vi "gen random emmiters.vi"(10 "rand limits":T14={"DOA range "={1634128.9560392164, 2964508.639841233}, "modulation depth"={67532.40039072247, 205475.5312375231}, "num of hoopers"=10, "num of frequncyes"={2, 1}, "QPSK"=TRUE, "BPSK"=TRUE, "LFM"=TRUE, "CW"=TRUE, "     f band range"={-77296466.97388633, 78525345.62211981}, "D.C range"={0.5407066052227343, 0.5038402457757296}, "hop rate range"={2.0915680786684536, 3.1385684721559217}, "span range "={1634128.9560392164, 2964508.639841233}, "amp range"={-21.121351766513058, -25.88325652841782}, "start time (sec)"=0.0, "end time (sec)"=50.0} {"start time (sec)" format="%#_13g"; "amp range" scale=0.0..-50.0 scale format="%#_g dB"; "span range" scale=1000000.0..30000000.0 scale format="%#_6p Hz"; "hop rate range" scale=1.0..3000.0 scale format="%#_6p"; "D.C range" scale=0.0..1.0; "f band range" scale=-1600000000.0..1600000000.0 scale format="%#_6p Hz"; "num of frequncyes" scale=1.0..300.0; "num of hoopers" scale=0.0..200.0; "modulation depth" scale=10000.0..30000000.0 scale format="%#_6p Hz"; "DOA range" scale=0.0..360.0 scale format="%#_6p deg"}, 11 "secnario config":T1={"devicess 2"=["IF_transiver_1", "IF_transiver_2"], "file paths"=[path "C:/Users/PXIe8108_Demo/Documents/CHAIM DATA/chaim/5785_sync_for_elbit/data/pdw_test_file.tdms", path "C:/Users/PXIe8108_Demo/Documents/CHAIM DATA/chaim/5785_sync_for_elbit/data/pdw_test_file.tdms", path "C:/Users/PXIe8108_Demo/Documents/CHAIM DATA/chaim/5785_sync_for_elbit/data/pdw_test_file.tdms", path "C:/Users/PXIe8108_Demo/Documents/CHAIM DATA/chaim/5785_sync_for_elbit/data/pdw_test_file.tdms"], "buffer size"=524288, "Fs  FPGA"=200000000.0, "SPC"=16.0, "center frequency (Hz) "=1000000000.0, "t clock ref"=[], "fpga rfe"=[], "tdms refs"=[], "niUsrpRio Session (out)"={"FPGA Interface"=refnum, "RIO Interface Number"=0, "Data Clock Rate"=0, "FPGA Data Clock Rate"=0, "Global Settings Register Bus"=refnum, "Radio 0 Settings Register Bus"=refnum, "Radio 1 Settings Register Bus"=refnum, "Radio Settings Bus Semaphore"=refnum, "DB Queues"=[], "Characterization Data Valid?"=FALSE, "EEPROM Header"={"Checksum"=0, "Product Code"=0, "Hardware Current Version"=0, "Hardware Oldest Compatible Version"=0, "EEPROM Map Current Version"=0, "EEPROM Map Oldest Compatible Version"=0, "User Password"="", "Pointer to Factory Header"=0, "Pointer to User Header"=0, "Recommended Interval"=0, "Number of Reserved Bytes"=9, "Number of Daughterboards"=0, "Daughterboard IDs"=[], "Daughterboard Serial Numbers"=[]}, "Device Data Header"={"Checksum"=0, "Number of Channels"=0, "Number of Gain Settings"=[], "Pointer to Characterization Data"=[], "Number of Reserved Bytes"=27, "Number of Frequencies"=[]}, "EEPROM Characterization Header"={"Checksum"=0, "Date"=timestamp(0 s since 1904-01-01), "Temperature"=0.0, "Misc. Info"="", "Pointer to Device Data Header"=0, "Number of Reserved Bytes"=28}, "Characterization Data"=[], "FPGA Current Version"=0, "FPGA Oldest Compatible Version"=0, "Fixed Logic Current Version"=0, "Fixed Logic Oldest Compatible Version"=0, "FPGA Radio Settings Bus Current Version"=0, "FPGA Radio Settings Bus Oldest Compatible Version"=0, "FPGA Board Config Current Version"=0, "FPGA Board Config Oldest Compatible Version"=0, "Daughterboard Clock Rate"=0, "daughterboard configuration session handles"=[]}, "RF gain "=10, "mode"=0, "vst_device"=[], "IQ_rare_p2p"=200000000.0, "stream sesion P2P"=[]} {"mode" scale=0.0..2.0; "RF gain" min=0 max=31 step=1; "niUsrpRio Session (out)"."Daughterboard Clock Rate" format="%#.3pHz"; "niUsrpRio Session (out)"."FPGA Data Clock Rate" format="%#.3pHz"; "niUsrpRio Session (out)"."Data Clock Rate" format="%#.3pHz"; "niUsrpRio Session (out)"."Characterization Data"."Frequencies [Hz]" format="%#_6p"; "niUsrpRio Session (out)"."EEPROM Characterization Header"."Pointer to Device Data Header" format="%x"; "niUsrpRio Session (out)"."EEPROM Characterization Header"."Checksum" format="%x"; "niUsrpRio Session (out)"."Device Data Header"."Pointer to Characterization Data" format="%x"; "niUsrpRio Session (out)"."Device Data Header"."Checksum" format="%x"; "niUsrpRio Session (out)"."EEPROM Header"."Pointer to User Header" format="%x"; "niUsrpRio Session (out)"."EEPROM Header"."Pointer to Factory Header" format="%x"; "niUsrpRio Session (out)"."EEPROM Header"."Product Code" format="%x"; "niUsrpRio Session (out)"."EEPROM Header"."Checksum" format="%x"; "center frequency (Hz)" format="%#.8p"; "buffer size" step=512}) -> (3 "Array":T12[](array[typedef]) {"t end" format="%#_3p"; "t start" format="%#_3p"; "DOA" format="%#_3p"; "mod depth" format="%#_3p"})   [LabVIEW 2021]
uses:
  random_limits.ctl
  emitter params.ctl
  mode_type.ctl
  secnario config.ctl
  <vilib>/userdefined/High Color/nirio_resource_hc.ctl
  <instrlib>/niUsrpRio/Config/v1/Host/Public/niUsrpRio Session.ctl
  <instrlib>/_niInstr/Register Bus/v0/Host/Public/Register Bus Session.ctl
  <instrlib>/_niInstr/Register Bus/v0/Host/Private/Session Data.ctl
  <instrlib>/niUsrpRio/Config/v1/Host/Private/DB Queue Reference.ctl
  <instrlib>/niUsrpRio/Config/v1/Host/Private/Daughterboard Data.ctl
  <instrlib>/niUsrpRio/Config/v1/Host/Private/ATR state data.ctl
  <instrlib>/niUsrpRio/Config/v1/Host/Private/Antenna Configuration.ctl
  <instrlib>/niUsrpRio/Config/v1/Host/Private/CPLD Power Mode.ctl
  <instrlib>/niUsrpRio/Config/v1/Host/Public/EEPROM Header.ctl
  <instrlib>/niUsrpRio/Config/v1/Host/Public/EEPROM Device Data Header.ctl
  <instrlib>/niUsrpRio/Config/v1/Host/Public/EEPROM Characterization Header.ctl
  <instrlib>/niUsrpRio/Config/v1/Host/Public/Characterization Data.ctl
  <instrlib>/niUsrpRio/Config/v1/Host/Public/IQ Imbalance.ctl
  <vilib>/numeric/Random Number (Range) DBL.vi
  <vilib>/numeric/Random Number (Range) U64.vi
  <vilib>/numeric/sub_Random U32.vi
  <instrlib>/_niInstr/Register Bus/v0/Host/niInstr Register Bus v0 Host.lvlib
  <instrlib>/niUsrpRio/Config/v1/Host/niUsrpRio Config v1 Host.lvlib
panel:
  # "available modulations:"
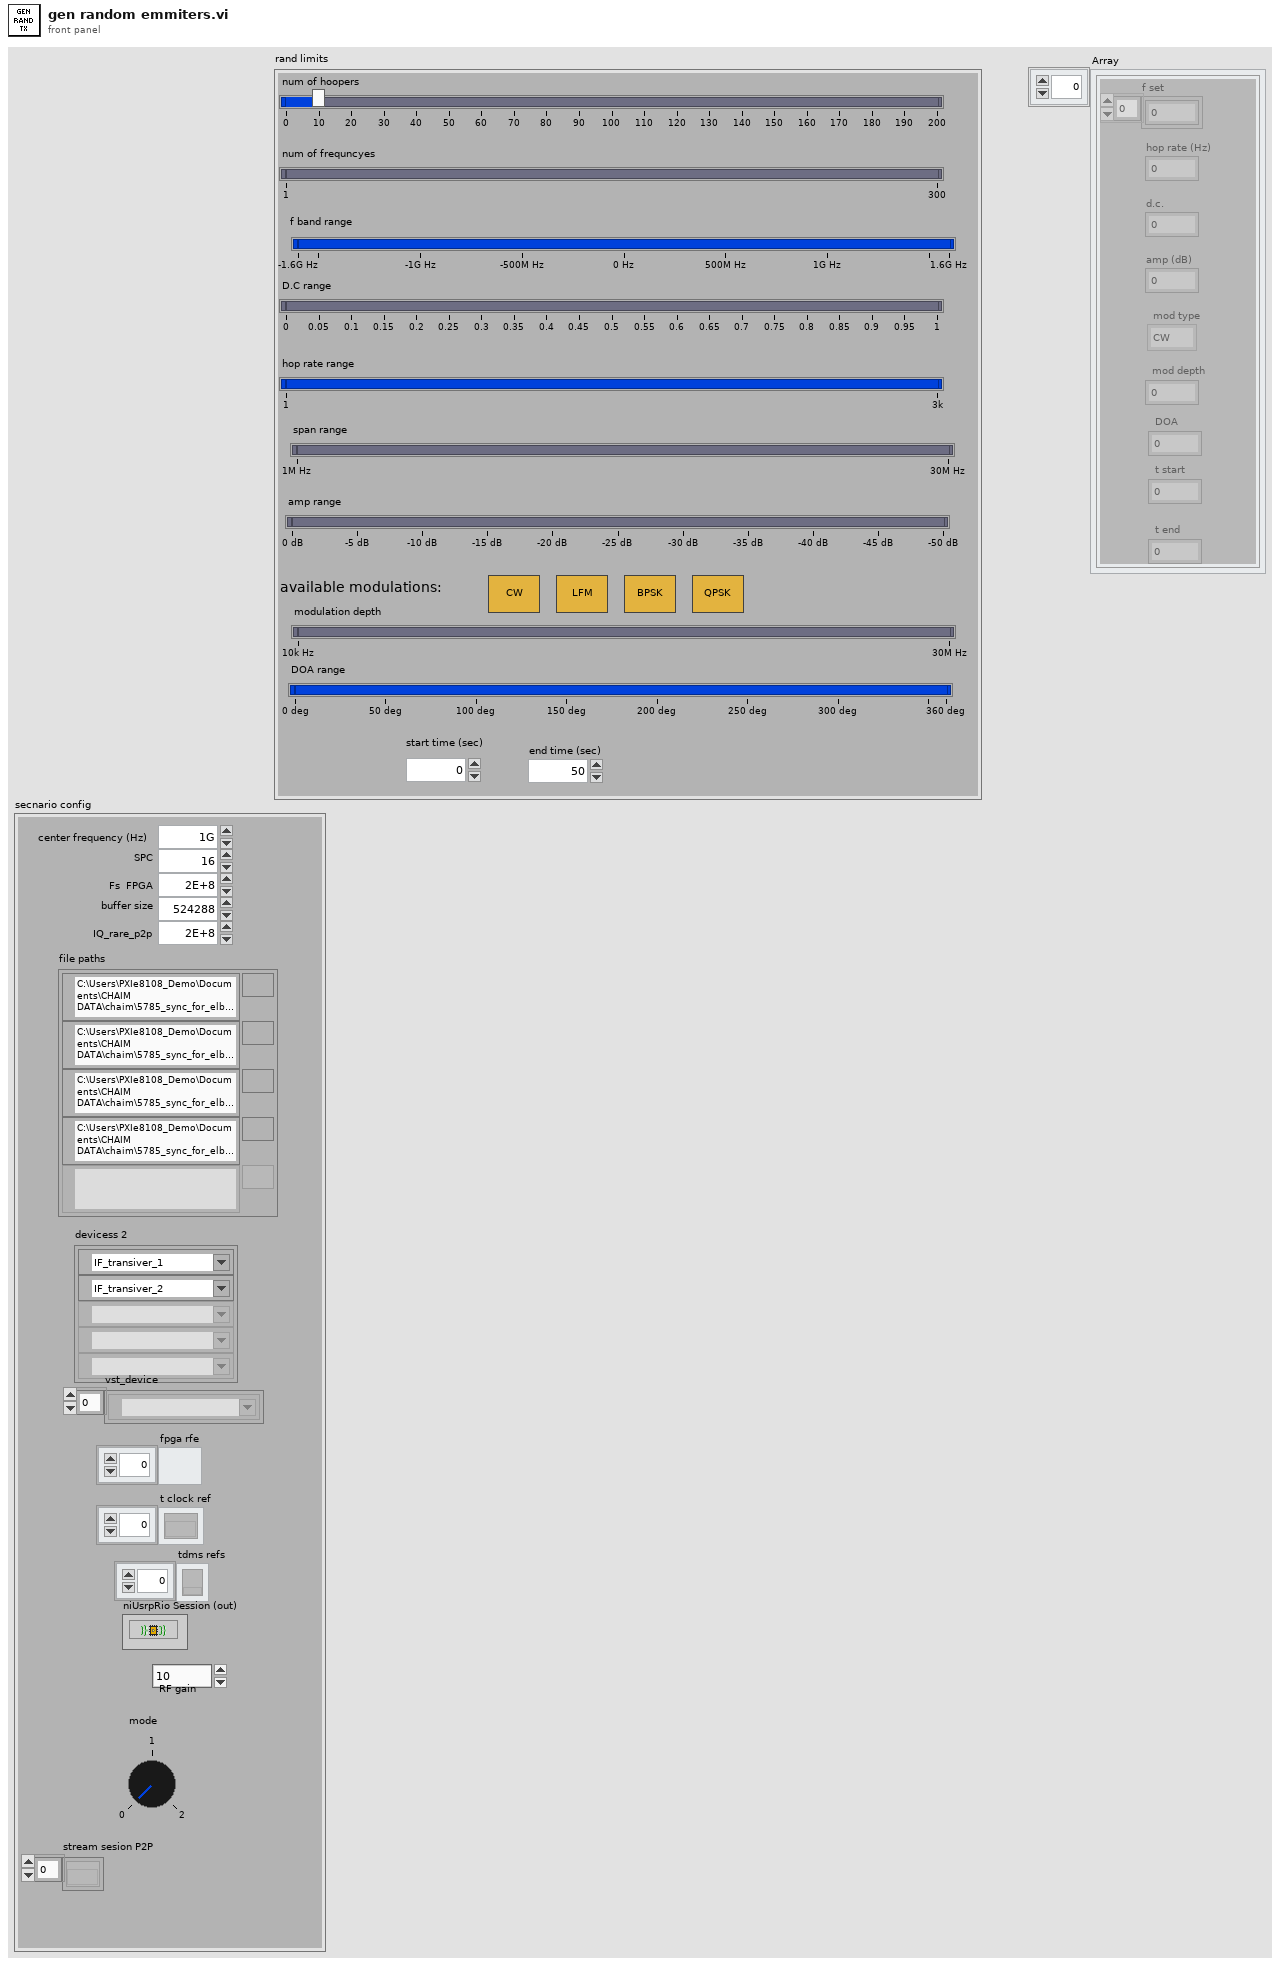
[diagram p1: front panel]
types:
  T1 = typedef "secnario config.ctl" = cluster{"devicess 2":T2[], "file paths":path[], "buffer size":u32, "Fs  FPGA":dbl, "SPC":dbl, "center frequency (Hz) ":dbl, "t clock ref":refnum<k20>[], "fpga rfe":refnum<k20>[], "tdms refs":refnum<k34>[], "niUsrpRio Session (out)":T3, "RF gain ":i32, "mode":u8, "vst_device":refnum<k15>[], "IQ_rare_p2p":dbl, "stream sesion P2P":refnum<k20>[]}
  T2 = typedef "nirio_resource_hc.ctl" = tag
  T3 = typedef "niUsrpRio Config v1 Host.lvlib/niUsrpRio Session.ctl" = cluster{"FPGA Interface":refnum<k20>, "RIO Interface Number":u32, "Data Clock Rate":u32, "FPGA Data Clock Rate":u32, "Global Settings Register Bus":T4, "Radio 0 Settings Register Bus":T4, "Radio 1 Settings Register Bus":T4, "Radio Settings Bus Semaphore":T5, "DB Queues":T6[], "Characterization Data Valid?":bool, "EEPROM Header":T7, "Device Data Header":T8, "EEPROM Characterization Header":T9, "Characterization Data":T10[], "FPGA Current Version":u32, "FPGA Oldest Compatible Version":u32, "Fixed Logic Current Version":u32, "Fixed Logic Oldest Compatible Version":u32, "FPGA Radio Settings Bus Current Version":u32, "FPGA Radio Settings Bus Oldest Compatible Version":u32, "FPGA Board Config Current Version":u32, "FPGA Board Config Oldest Compatible Version":u32, "Daughterboard Clock Rate":u32, "daughterboard configuration session handles":u64[]}
  T4 = typedef "niInstr Register Bus v0 Host.lvlib/Register Bus Session.ctl" = refnum<queue>
  T5 = typedef "Semaphore RefNum" = refnum<k1>
  T6 = typedef "niUsrpRio Config v1 Host.lvlib/DB Queue Reference.ctl" = refnum<queue>
  T7 = typedef "niUsrpRio Config v1 Host.lvlib/EEPROM Header.ctl" = cluster{"Checksum":u32, "Product Code":u16, "Hardware Current Version":u16, "Hardware Oldest Compatible Version":u16, "EEPROM Map Current Version":u16, "EEPROM Map Oldest Compatible Version":u16, "User Password":string, "Pointer to Factory Header":u32, "Pointer to User Header":u32, "Recommended Interval":u16, "Number of Reserved Bytes":i32, "Number of Daughterboards":u8, "Daughterboard IDs":u16[], "Daughterboard Serial Numbers":string[]}
  T8 = typedef "niUsrpRio Config v1 Host.lvlib/EEPROM Device Data Header.ctl" = cluster{"Checksum":u32, "Number of Channels":u8, "Number of Gain Settings":u16[], "Pointer to Characterization Data":u32[], "Number of Reserved Bytes":i32, "Number of Frequencies":u16[]}
  T9 = typedef "niUsrpRio Config v1 Host.lvlib/EEPROM Characterization Header.ctl" = cluster{"Checksum":u32, "Date":timestamp, "Temperature":sgl, "Misc. Info":string, "Pointer to Device Data Header":u32, "Number of Reserved Bytes":i32}
  T10 = typedef "niUsrpRio Config v1 Host.lvlib/Characterization Data.ctl" = cluster{"Gains[dB]":dbl[], "Frequencies [Hz]":dbl[], "IQ Imbalance Table":T11[], "Measured Gains[dB]":dbl[][]}
  T11 = typedef "niUsrpRio Config v1 Host.lvlib/IQ Imbalance.ctl" = cluster{"Gain Imbalance [linear]":dbl, "Phase Imbalance [radians]":dbl, "Offset":cdb}
  T12 = typedef "emitter params.ctl" = cluster{"f set":dbl[], "hop rate (Hz)":dbl, "d.c.":dbl, "amp (dB)":dbl, "mod type":T13, "mod depth":dbl, "DOA":dbl, "t start":dbl, "t end":dbl}
  T13 = typedef "mode_type.ctl" = enum8{"CW", "NC - CW", "NC - cw", "LFM", "BPSK", "QPSK"}
  T14 = typedef "random_limits.ctl" = cluster{"DOA range ":cluster{dbl, dbl}, "modulation depth":cluster{dbl, dbl}, "num of hoopers":i32, "num of frequncyes":cluster{i32, i32}, "QPSK":bool, "BPSK":bool, "LFM":bool, "CW":bool, "     f band range":cluster{dbl, dbl}, "D.C range":cluster{dbl, dbl}, "hop rate range":cluster{dbl, dbl}, "span range ":cluster{dbl, dbl}, "amp range":cluster{dbl, dbl}, "start time (sec)":dbl, "end time (sec)":dbl}
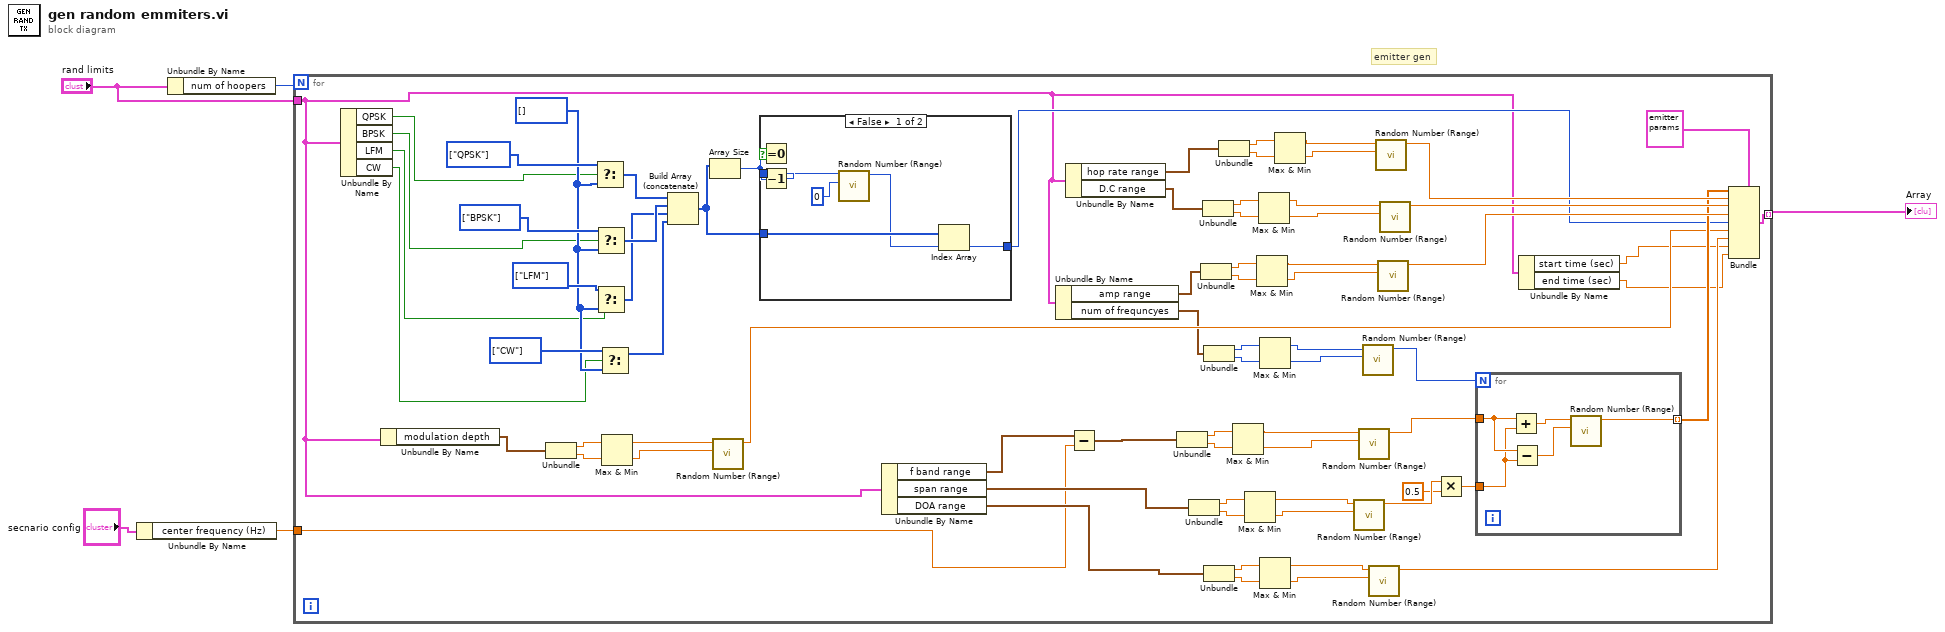
[diagram p0: block diagram]
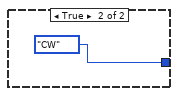
[diagram p2: hidden frame]
diagram:
  # "emitter gen"
  n1 = Unbundle By Name("secnario config") -> ("center frequency (Hz)"=w1:dbl)
  n2 = Unbundle By Name("rand limits") -> ("num of hoopers"=w4:i32)
  n3 = for {
    N: w4 -> [_]
    tunnel: [w72] -> w5 mode=indexing
    tunnel: "rand limits" -> [w10]
    tunnel: w1 -> [w7]
    w32 = T13[] [enum."QPSK"] items=["CW", "NC - CW", "NC - cw", "LFM", "BPSK", "QPSK"]
    w28 = T13[] [] items=["CW", "NC - CW", "NC - cw", "LFM", "BPSK", "QPSK"]
    w31 = T13[] [enum."BPSK"] items=["CW", "NC - CW", "NC - cw", "LFM", "BPSK", "QPSK"]
    w30 = T13[] [enum."LFM"] items=["CW", "NC - CW", "NC - cw", "LFM", "BPSK", "QPSK"]
    w29 = T13[] [enum."CW"] items=["CW", "NC - CW", "NC - cw", "LFM", "BPSK", "QPSK"]
    n4 = Unbundle By Name(w10) -> ("QPSK"=w22:bool, "BPSK"=w21:bool, "LFM"=w20:bool, "CW"=w19:bool)
    n5 = Unbundle By Name(w10) -> ("modulation depth"=w9:cluster{dbl, dbl})
    n6 = Unbundle(w9) -> (w46:dbl, w45:dbl)
    n7 = Select(t=w32, s=w22, f=w28) -> (s? t:f=w42:T13[])
    n8 = Select(t=w31, s=w21, f=w28) -> (s? t:f=w41:T13[])
    n9 = Select(t=w30, s=w20, f=w28) -> (s? t:f=w40:T13[])
    n10 = Select(t=w29, s=w19, f=w28) -> (s? t:f=w39:T13[])
    n11 = Max & Min(x=w46, y=w45) -> (max(x,y)=w44:dbl, min(x,y)=w43:dbl)
    n12 = Build Array (concatenate)(w42, w41, w40, w39) -> (w38:T13[])
    n13 = Array Size(array=w38) -> (size(s)=w34:i32)
    n14 = call-poly <vilib>:"Random Number (Range).vi"("lower bound (0)"=w43, "upper bound (100)"=w44) -> ("number"=w35:dbl)  [unwired: 9 in]
    n15 = Equal To 0?(x=w34) -> (x = 0?=w36:bool)
    n16 = Decrement(x=w34) -> (x-1=w33:i32)
    n17 = case shown="False" w36 {
      tunnel: w38 -> [w85 _]
      tunnel: [w83 mode_type."CW" ("mod type")] -> w37
      tunnel: w33 -> [w82 _]
      frame False {
        n18 = call-poly <vilib>:"Random Number (Range).vi"("lower bound (0)"=u64 0, "upper bound (100)"=w82) -> ("number"=w84:u64)  [unwired: 9 in]
        n19 = Index Array(array=w85, index=w84) -> (element=w83:T13)
      }
      frame True {
      }
    }
    n20 = Unbundle By Name(w10) -> ("f band range"=w8:cluster{dbl, dbl}, "span range"=w13:cluster{dbl, dbl}, "DOA range"=w14:cluster{dbl, dbl})
    n21 = Unbundle By Name(w10) -> ("amp range"=w16:cluster{dbl, dbl}, "num of frequncyes"=w15:cluster{i32, i32})
    n22 = Unbundle By Name(w10) -> ("hop rate range"=w18:cluster{dbl, dbl}, "D.C range"=w17:cluster{dbl, dbl})
    n23 = Subtract(x=w8, y=w7) -> (x-y=w6:cluster{dbl, dbl})
    n24 = Unbundle(w6) -> (w54:dbl, w53:dbl)
    n25 = Unbundle(w13) -> (w49:dbl, w50:dbl)
    n26 = Unbundle(w16) -> (w68:dbl, w67:dbl)
    n27 = Unbundle(w17) -> (w65:dbl, w66:dbl)
    n28 = Unbundle(w15) -> (w57:i32, w58:i32)
    n29 = Unbundle(w14) -> (w25:dbl, w24:dbl)
    n30 = Unbundle(w18) -> (w62:dbl, w61:dbl)
    n31 = Max & Min(x=w54, y=w53) -> (max(x,y)=w52:dbl, min(x,y)=w51:dbl)
    n32 = Max & Min(x=w49, y=w50) -> (max(x,y)=w48:dbl, min(x,y)=w47:dbl)
    n33 = Max & Min(x=w68, y=w67) -> (max(x,y)=w70:dbl, min(x,y)=w69:dbl)
    n34 = Max & Min(x=w65, y=w66) -> (max(x,y)=w64:dbl, min(x,y)=w63:dbl)
    n35 = Max & Min(x=w57, y=w58) -> (max(x,y)=w56:i32, min(x,y)=w55:i32)
    n36 = Max & Min(x=w25, y=w24) -> (max(x,y)=w26:dbl, min(x,y)=w27:dbl)
    n37 = Max & Min(x=w62, y=w61) -> (max(x,y)=w60:dbl, min(x,y)=w59:dbl)
    n38 = call-poly <vilib>:"Random Number (Range).vi"("lower bound (0)"=w47, "upper bound (100)"=w48) -> ("number"=w77:dbl)  [unwired: 9 in]
    n39 = call-poly <vilib>:"Random Number (Range).vi"("lower bound (0)"=w51, "upper bound (100)"=w52) -> ("number"=w75:dbl)  [unwired: 9 in]
    n40 = call-poly <vilib>:"Random Number (Range).vi"("lower bound (0)"=w55, "upper bound (100)"=w56) -> ("number"=w71:u64)  [unwired: 9 in]
    n41 = call-poly <vilib>:"Random Number (Range).vi"("lower bound (0)"=w27, "upper bound (100)"=w26) -> ("number"=w23:dbl)  [unwired: 9 in]
    n42 = call-poly <vilib>:"Random Number (Range).vi"("lower bound (0)"=w59, "upper bound (100)"=w60) -> ("number"=w80:dbl)  [unwired: 9 in]
    n43 = call-poly <vilib>:"Random Number (Range).vi"("lower bound (0)"=w69, "upper bound (100)"=w70) -> ("number"=w78:dbl)  [unwired: 9 in]
    n44 = call-poly <vilib>:"Random Number (Range).vi"("lower bound (0)"=w63, "upper bound (100)"=w64) -> ("number"=w79:dbl)  [unwired: 9 in]
    n45 = Multiply(x=w77, y=0.5) -> (x*y=w74:dbl)
    n46 = for {
      N: w71 -> [_]
      tunnel: w75 -> [w92]
      tunnel: w74 -> [w91]
      tunnel: [w88] -> w73 mode=indexing
      n47 = Add(x=w92, y=w91) -> (x+y=w89:dbl)
      n48 = Subtract(x=w92, y=w91) -> (x-y=w90:dbl)
      n49 = call-poly <vilib>:"Random Number (Range).vi"("lower bound (0)"=w90, "upper bound (100)"=w89) -> ("number"=w88:dbl)  [unwired: 9 in]
    }
    n50 = Unbundle By Name(w10) -> ("start time (sec)"=w12:dbl, "end time (sec)"=w11:dbl)
    n51 = Bundle(cluster=T12 {"f set"=[1000000.0], "hop rate (Hz)"=300000.0, "d.c."=0.0, "amp (dB)"=-20.0, "mod type"=enum."CW", "mod depth"=0.0, "DOA"=0.0, "t start"=0.0, "t end"=0.0} ("Cluster"), "f set"=w73, "hop rate (Hz)"=w80, "d.c."=w79, "amp (dB)"=w78, "mod type"=w37, "mod depth"=w35, "DOA"=w23, "t start"=w12, "t end"=w11) -> (w72:T12)
  }
  "Array" <- w5
